vi "Connection Updated.vi"(8 "error in":errorcluster, 9 "Key":string, 10 "Connection State":bool) -> (0 "error out":errorcluster)   [LabVIEW 2024, in "IOLink.lvlib"]
doc: "Lets listeners know that the connection state of the io link master has been updated\n_____\nCreated using DQMH Event Scripter 7.0.0.1280."
uses:
  IOLink.lvlib
  Connection Updated Argument--cluster.ctl
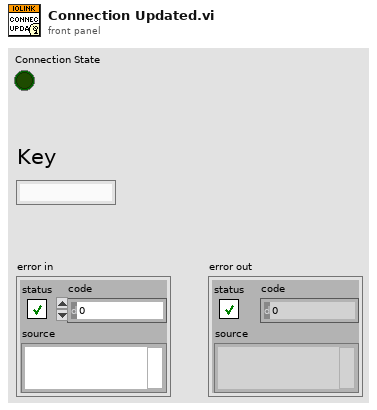
[diagram p1: front panel]
types:
  T1 = typedef "IOLink.lvlib/Connection Updated Argument--cluster.ctl" = cluster{"Connection State":bool, "Key":string}
  T2 = typedef "IOLink.lvlib/Broadcast Events--cluster.ctl" = cluster{"Module Did Init":refnum<user-event>, "Status Updated":refnum<user-event>, "Error Reported":refnum<user-event>, "Module Did Stop":refnum<user-event>, "Update Module Execution Status":refnum<user-event>, "Data Updated":refnum<user-event>, "Connection Updated":refnum<user-event>}
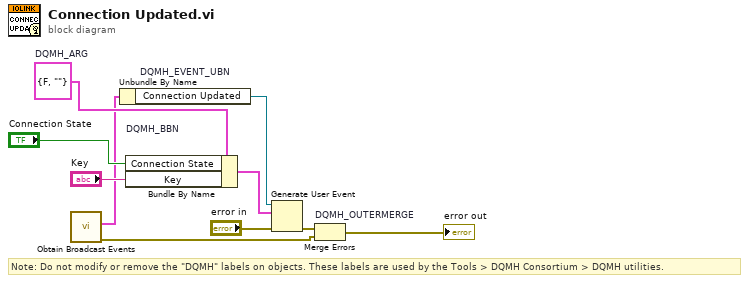
[diagram p0: block diagram]
diagram:
  w5 = T1 {"Connection State"=FALSE, "Key"=""}  # DQMH_ARG
  # "Note: Do not modify or remove the \"DQMH\" labels on objects. These labels are used by the Tools > DQMH Consortium > DQMH utilities."
  n1 = call "Obtain Broadcast Events.vi"() -> ("error out"=w2:errorcluster, "IOLink Broadcast Events"=w1:T2)  [unwired: 10 in]
  n2 = Unbundle By Name "DQMH_EVENT_UBN"(w1) -> ("Connection Updated"=w7:refnum<user-event>)
  n3 = Bundle By Name "DQMH_BBN"(cluster=w5, "Connection State"="Connection State", "Key"="Key") -> (w8:T1)
  n4 = Generate User Event(user event=w7, event data cluster=w8, error in="error in") -> (error out=w6:errorcluster)  [unwired: 1 in, 1 out]
  n5 = Merge Errors "DQMH_OUTERMERGE"(w6, w2) -> (→"error out":errorcluster)
